vi "LV SciSDK LIST STOP.vi"(8 "error in (no error)":errorcluster, 9 "List Handle In":T1) -> (0 "error out":errorcluster, 1 "List Handle Out":T1, 3 "function return":i32)   [LabVIEW 2021]
uses:
  SciSDK_Labview.lvlib
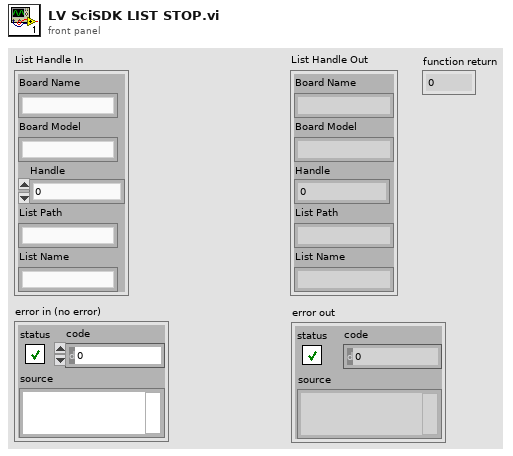
[diagram p1: front panel]
types:
  T1 = cluster{"Board Name":string, "Board Model":string, "Handle":u64, "List Path":string, "List Name":string}
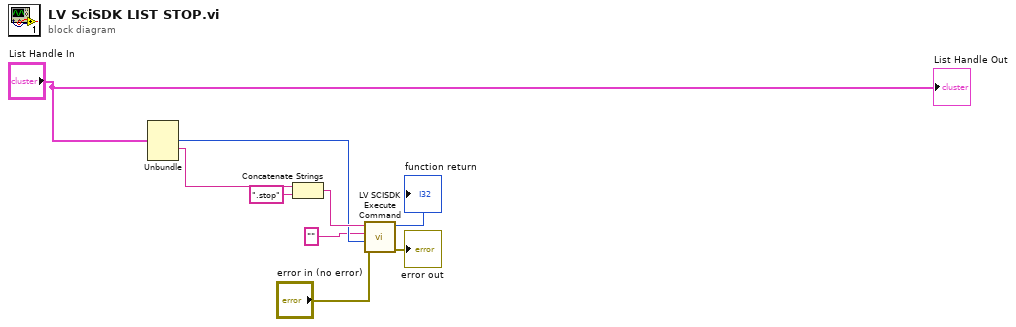
[diagram p0: block diagram]
diagram:
  n1 = Unbundle("List Handle In") -> ("Handle"=w5:u64, "List Path"=w8:string)  [unwired: 3 out]
  n2 = Concatenate Strings(w8, ".stop" ("string")) -> (w6:string)
  n3 = call "LV SCISDK Execute Command.vi"("error in (no error)"="error in (no error)", "handle"=w5, "value"="", "Path"=w6) -> ("error out"=→"error out":errorcluster, "function return"=→"function return":i32)  [unwired: 5 in, 1 out]
  "List Handle Out" <- "List Handle In"
